vi "ParseDescription.vi"(11 "Descrition":string) -> (2 "Submit tokens":string[](array[string]), 3 "Filtered Description":string)   [LabVIEW 2014, in "BooleanControl.lvclass"]
uses:
  BooleanControl.lvclass
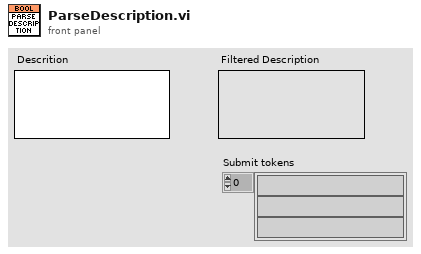
[diagram p1: front panel]
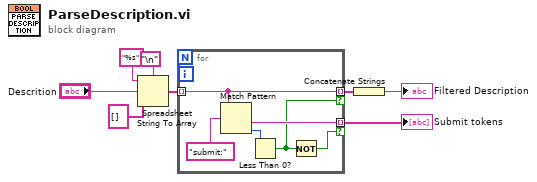
[diagram p0: block diagram]
diagram:
  n1 = Spreadsheet String To Array(delimiter (Tab)="\n", format string="%s", spreadsheet string="Descrition", array type (2D Dbl)=string[] []) -> (array=w4:string[])
  n2 = for {
    tunnel: w4 -> [w13] mode=indexing
    tunnel: [w13] -> w3 mode=indexing if=w10
    tunnel: [w11] -> w1 mode=indexing if=w9
    n3 = Match Pattern(string=w13, regular expression="submit:" ("format string")) -> (after substring=w11:string, offset past match=w12:i32)  [unwired: 1 in, 2 out]
    n4 = Less Than 0?(x=w12) -> (x < 0?=w10:bool)
    n5 = Not(x=w10) -> (.not. x?=w9:bool)
  }
  "Submit tokens" <- w1
  n6 = Concatenate Strings(w3) -> (→"Filtered Description":string)
